vi "SubViTestGlobals.vi"() -> ()   [LabVIEW 2014]
panel:
  in  "stop":bool
  out "insideloop":i32
  out "0notPressed1Pressed":i16
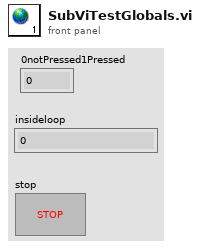
[diagram p1: front panel]
diagram:
